vi "Control Camera Properties.vi"(8 "error in (no error)":errorcluster, 10 "Control Camera Properties":T3={"Packet Size"=1500, "Pixel Format"=17825797, "Gain in dB"=1.0, "Exposure Time in µs"=1500, "Stream MBytes per Second"=124} {"Stream MBytes per Second" min=1 max=124 step=1 format="%#.6p"; "Exposure Time in µs" min=21 max=153391689 format="%#.0f"; "Gain in dB" min=0.0 max=26.0 format="%#_2g"; "Pixel Format" items=["Mono 12 Packed"=17563654, "Mono 12"=17825797, "Mono 8"=17301505]}, 11 "IMAQdx Session":T2) -> (0 "error out 2":errorcluster, 2 "output cluster":T1, 3 "Session Out 2":T2)   [LabVIEW 2014]
uses:
  <vilib>/userdefined/High Color/IMAQdx.ctl
  type definitions/control camera properties.ctl
  <resource>/objmgr/imaqdx.rc
panel:
  # "Bytes"
  # "Trigger"
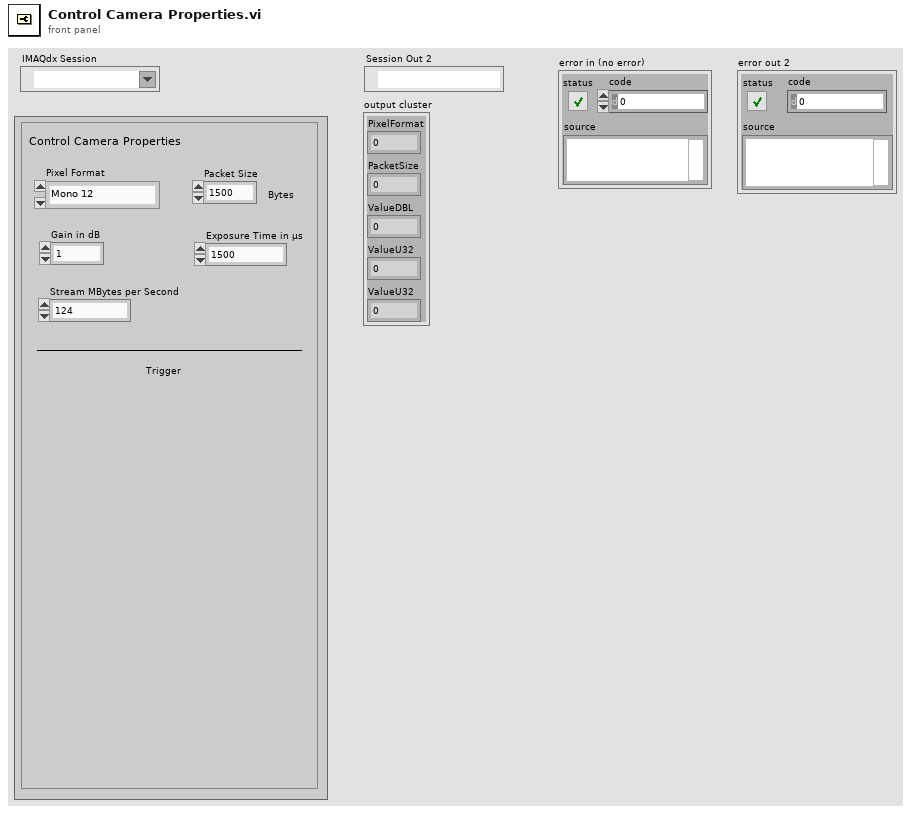
[diagram p1: front panel]
types:
  T1 = cluster{"PixelFormat":u32, "PacketSize":u32, "ValueDBL":dbl, "ValueU32":u32, "ValueU32":u32}
  T2 = typedef "IMAQdx.ctl" = refnum<k21>
  T3 = typedef "control camera properties.ctl" = cluster{"Packet Size":u32, "Pixel Format":u32, "Gain in dB":dbl, "Exposure Time in µs":u32, "Stream MBytes per Second":u32}
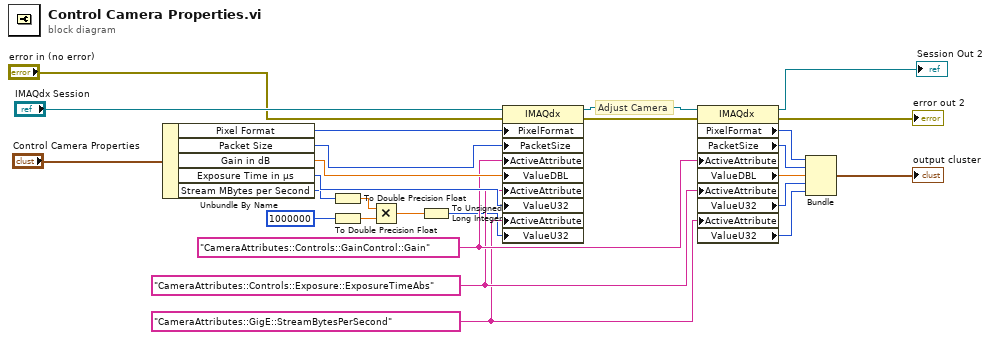
[diagram p0: block diagram]
diagram:
  w9 = "CameraAttributes::GigE::StreamBytesPerSecond"
  w17 = "CameraAttributes::Controls::Exposure::ExposureTimeAbs"
  w18 = "CameraAttributes::Controls::GainControl::Gain"
  # "Adjust Camera"
  n1 = Unbundle By Name("Control Camera Properties") -> ("Pixel Format"=w24:u32, "Packet Size"=w23:u32, "Gain in dB"=w22:dbl, "Exposure Time in µs"=w21:u32, "Stream MBytes per Second"=w2:u32)
  n2 = To Double Precision Float(number=w2) -> (double precision float=w8:dbl)
  n3 = To Double Precision Float(number=u32 1000000 ("y")) -> (double precision float=w7:dbl)
  n4 = Multiply(x=w8, y=w7) -> (x*y=w6:dbl)
  n5 = To Unsigned Long Integer(number=w6) -> (unsigned 32bit integer=w3:u32)
  n6 = property class="IMAQdx"(reference="IMAQdx Session", error in="error in (no error)", "PixelFormat"=w24, "PacketSize"=w23, "ActiveAttribute"=w18, "ValueDBL"=w22, "ActiveAttribute"=w17, "ValueU32"=w21, "ActiveAttribute"=w9, "ValueU32"=w3) -> (reference out=w19:T2, error out=w12:errorcluster)
  n7 = property class="IMAQdx"(reference=w19, error in=w12, "ActiveAttribute"=w18, "ActiveAttribute"=w17, "ActiveAttribute"=w9) -> (reference out=→"Session Out 2":T2, error out=→"error out 2":errorcluster, "PixelFormat"=w16:u32, "PacketSize"=w15:u32, "ValueDBL"=w14:dbl, "ValueU32"=w13:u32, "ValueU32"=w5:u32)
  n8 = Bundle("PixelFormat"=w16, "PacketSize"=w15, "ValueDBL"=w14, "ValueU32"=w13, "ValueU32"=w5) -> (→"output cluster":T1)  [unwired: 1 in]
